vi "Day02-05_파일IO, TDMS.vi"() -> ()   [LabVIEW 2021]
uses:
  <vilib>/Utility/sysdir.llb/System Directory Type.ctl
  <vilib>/Utility/file.llb/Read Delimited Spreadsheet (DBL).vi
  <vilib>/Utility/file.llb/Write Delimited Spreadsheet (DBL).vi
panel:
  out "출력 데이터":dbl[][](array[numeric]) caption="모든 행"
  out "추가된 경로 3":path
  out "system directory 4":path caption="시스템 디렉토리"
  out "추가된 경로 2":path
  out "system directory 3":path caption="시스템 디렉토리"
  out "데이터":dbl[](array[numeric])
  out "데이터 2":string[][](array[string])
  out "system directory 2":path caption="시스템 디렉토리"
  out "추가된 경로":path
  out "system directory":path caption="시스템 디렉토리"
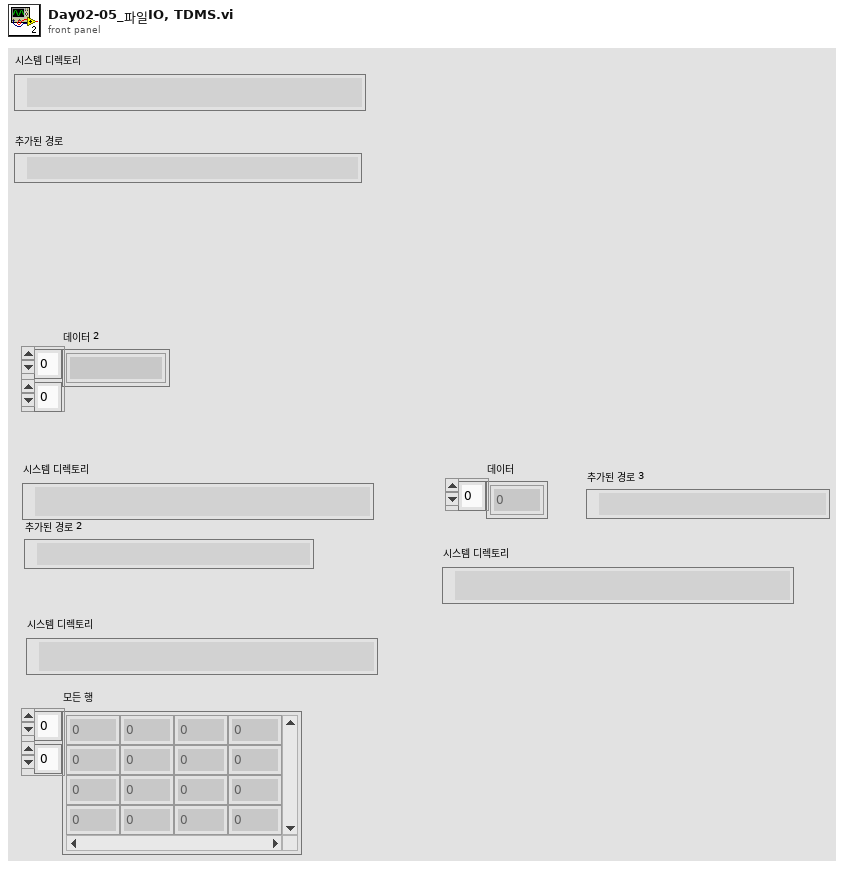
[diagram p1: front panel]
types:
  T1 = typedef "System Directory Type.ctl" = i32
  T2 = enum16{"open", "replace", "create", "open or create", "replace or create", "replace or create with confirmation"}
  T3 = enum16{"open", "open or create", "create or replace", "create", "open (read-only)"}
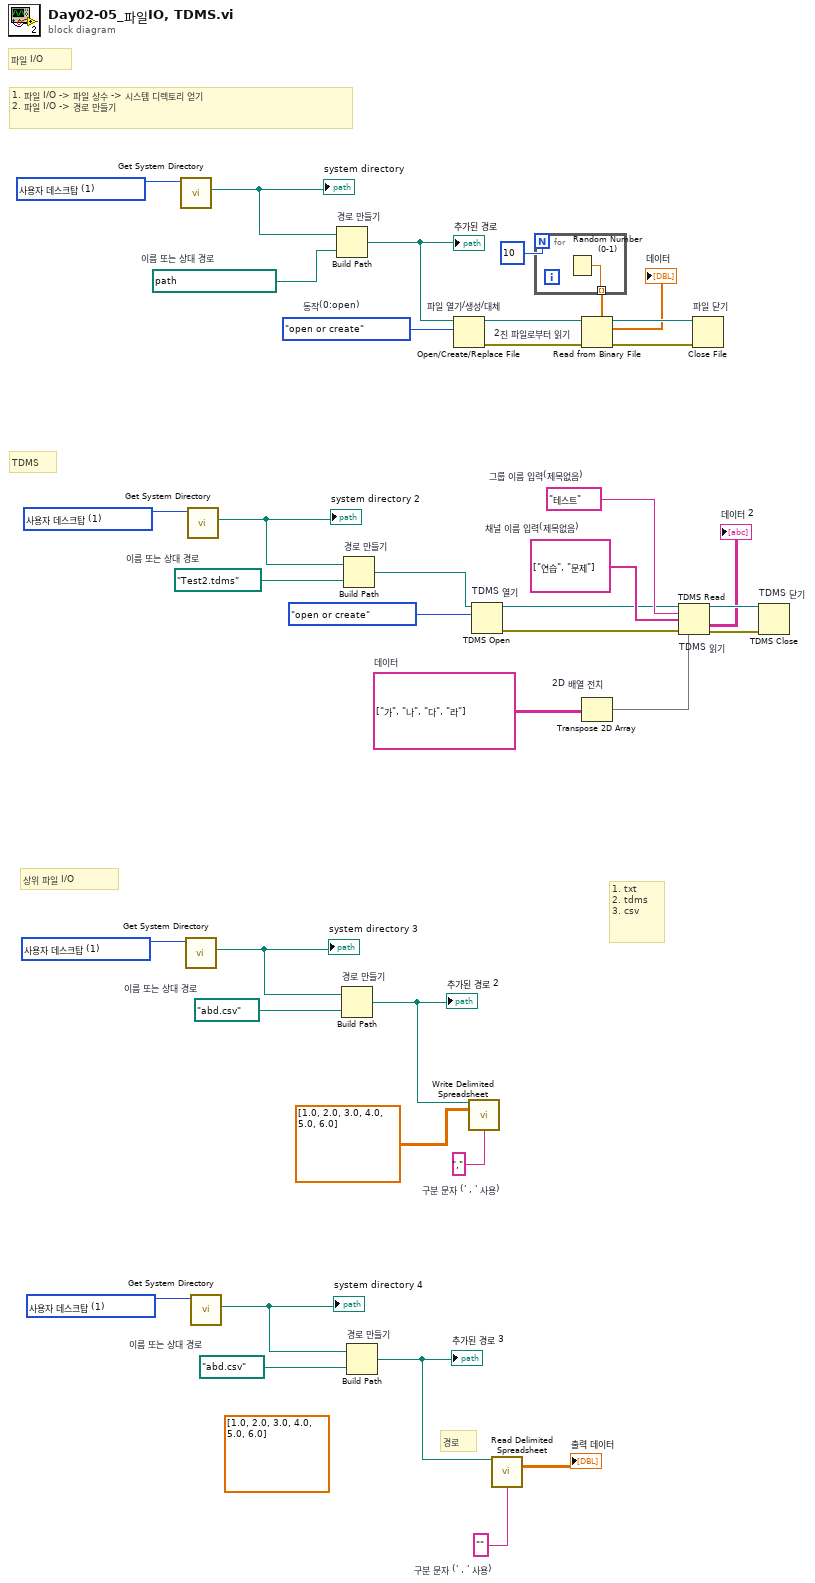
[diagram p0: block diagram]
diagram:
  w1 = ","  # 구분 문자 (' , ' 사용)
  w6 = path "abd.csv"  # 이름 또는 상대 경로
  w4 = T1 1 items=["사용자 홈"=0, "사용자 데스크탑"=1, "사용자 문서"=2, "사용자 어플리케이션 데이터"=3, "사용자 환경"=4, "사용자 임시"=5, "퍼블릭 문서"=6, "퍼블릭 어플리케이션 데이터"=7, "퍼블릭 환경"=8, "퍼블릭 캐시"=13, "시스템 코어 라이브러리"=9, "시스템 설치된 라이브러리"=10, "어플리케이션 파일"=11, "부팅 볼륨 루트"=12] ("system directory type")
  w14 = T2."open or create"  # 동작(0:open)
  w16 = path "2진파일 쓰기.txt"  # 이름 또는 상대 경로
  w18 = T1 1 items=["사용자 홈"=0, "사용자 데스크탑"=1, "사용자 문서"=2, "사용자 어플리케이션 데이터"=3, "사용자 환경"=4, "사용자 임시"=5, "퍼블릭 문서"=6, "퍼블릭 어플리케이션 데이터"=7, "퍼블릭 환경"=8, "퍼블릭 캐시"=13, "시스템 코어 라이브러리"=9, "시스템 설치된 라이브러리"=10, "어플리케이션 파일"=11, "부팅 볼륨 루트"=12] ("system directory type")
  w19 = ""  # 구분 문자 (' , ' 사용)
  (unwired) dbl[][] [[1.0, 2.0, 3.0], [4.0, 5.0, 6.0]]
  w24 = path "abd.csv"  # 이름 또는 상대 경로
  w22 = T1 1 items=["사용자 홈"=0, "사용자 데스크탑"=1, "사용자 문서"=2, "사용자 어플리케이션 데이터"=3, "사용자 환경"=4, "사용자 임시"=5, "퍼블릭 문서"=6, "퍼블릭 어플리케이션 데이터"=7, "퍼블릭 환경"=8, "퍼블릭 캐시"=13, "시스템 코어 라이브러리"=9, "시스템 설치된 라이브러리"=10, "어플리케이션 파일"=11, "부팅 볼륨 루트"=12] ("system directory type")
  w33 = string[][] [["가", "나"], ["다", "라"]]  # 데이터
  w30 = string[] ["연습", "문제"]  # 채널 이름 입력(제목없음)
  w29 = "테스트"  # 그룹 이름 입력(제목없음)
  w38 = path "Test2.tdms"  # 이름 또는 상대 경로
  w36 = T1 1 items=["사용자 홈"=0, "사용자 데스크탑"=1, "사용자 문서"=2, "사용자 어플리케이션 데이터"=3, "사용자 환경"=4, "사용자 임시"=5, "퍼블릭 문서"=6, "퍼블릭 어플리케이션 데이터"=7, "퍼블릭 환경"=8, "퍼블릭 캐시"=13, "시스템 코어 라이브러리"=9, "시스템 설치된 라이브러리"=10, "어플리케이션 파일"=11, "부팅 볼륨 루트"=12] ("system directory type")
  # "1. txt\n2. tdms\n3. csv"
  # "상위 파일 I/O"
  # "1. 파일 I/O -> 파일 상수 -> 시스템 디렉토리 얻기\n2. 파일 I/O -> 경로 만들기"
  # "파일 I/O"
  # "경로"
  # "TDMS"
  n1 = call <vilib>:"Get System Directory.vi"("system directory type"=w18) -> ("system directory"=w17:path)  [unwired: 10 in]
  "system directory" <- w17
  n2 = call <vilib>:"Get System Directory.vi"("system directory type"=w4) -> ("system directory"=w5:path)  [unwired: 10 in]
  "system directory 3" <- w5
  n3 = call <vilib>:"Get System Directory.vi"("system directory type"=w36) -> ("system directory"=w37:path)  [unwired: 10 in]
  "system directory 2" <- w37
  n4 = call <vilib>:"Get System Directory.vi"("system directory type"=w22) -> ("system directory"=w23:path)  [unwired: 10 in]
  "system directory 4" <- w23
  n5 = Build Path "경로 만들기"(base path=w17, name or relative path=w16) -> (appended path=w15:path)
  "추가된 경로" <- w15
  n6 = Build Path "경로 만들기"(base path=w5, name or relative path=w6) -> (appended path=w3:path)
  "추가된 경로 2" <- w3
  n7 = Build Path "경로 만들기"(base path=w37, name or relative path=w38) -> (appended path=w34:path)
  n8 = Build Path "경로 만들기"(base path=w23, name or relative path=w24) -> (appended path=w21:path)
  "추가된 경로 3" <- w21
  n9 = Open/Create/Replace File "파일 열기/생성/대체"(file path (use dialog)=w15, operation (0:open)=w14) -> (refnum out=w12:refnum<file>, error out=w9:errorcluster)  [unwired: 4 in, 1 out]
  n10 = call-poly <vilib>:"Write Delimited Spreadsheet.vi"("file path (dialog if empty)"=w3, "2D data"=dbl[][] [[1.0, 2.0, 3.0], [4.0, 5.0, 6.0]], "delimiter (\\t)"=w1) -> ()  [unwired: 11 in, 2 out]
  n11 = TDMS Open "TDMS 열기"(10:T3."open or create" ("동작(0:open)"), 11:w34) -> (0:w27:errorcluster, 3:w25:refnum<k34>)  [unwired: 5 in]
  n12 = call-poly <vilib>:"Read Delimited Spreadsheet.vi"("file path (dialog if empty)"=w21, "delimiter (\\t)"=w19) -> ("all rows"=→"출력 데이터":dbl[][])  [unwired: 8 in, 5 out]
  n13 = for {
    N: 10 -> [_]
    tunnel: [w39] -> w8 mode=indexing
    n14 = Random Number (0-1)() -> (number: 0 to 1=w39:dbl)
  }
  n15 = Read from Binary File "2진 파일로부터 읽기"(5:w8, 8:w9, 11:w12) -> (0:w10:errorcluster, 2:→"데이터":dbl[], 3:w11:refnum<file>)  [unwired: 3 in, 1 out]
  n16 = Transpose 2D Array "2D 배열 전치"(2D array=w33) -> (transposed array=w31:string[][])
  n17 = TDMS Read "TDMS 읽기"(0:w25, 5:w29, 7:w30, 11:w27, 12:w31) -> (4:w32:refnum<k34>, 10:→"데이터 2":string[][], 15:w26:errorcluster)  [unwired: 3 in, 3 out]
  n18 = Close File "파일 닫기"(refnum=w11, error in=w10) -> ()  [unwired: 2 out]
  n19 = TDMS Close "TDMS 닫기"(8:w26, 11:w32) -> ()  [unwired: 2 out]
